vi "Calculate_Subtrack_Properties-1.vi"(6 "error IN":errorcluster, 7 "[IN] Areas particles\nPrimary Detected":dbl[][](array[numeric]), 8 "[IN] Primary \n(X,Y) Detected":dbl[][](array[numeric]), 9 "[IN] Subtrack":T1) -> (0 "error OUT":errorcluster, 1 "[OUT] Length of track":u8, 2 "[OUT] Areas":dbl[](array[numeric]), 3 "[OUT] dR (displ)":dbl[](array[numeric]))   [LabVIEW 2013]
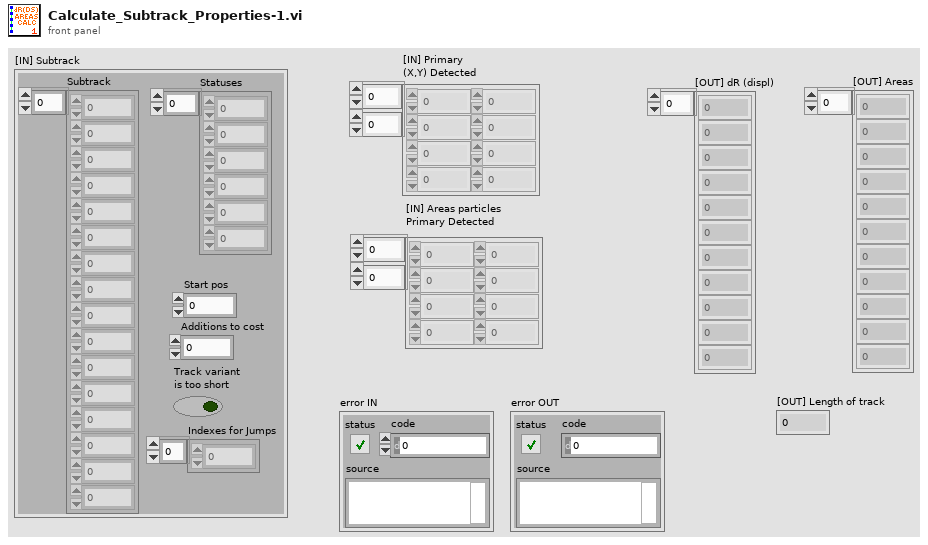
[diagram p1: front panel]
types:
  T1 = cluster{"Subtrack":dbl[], "Statuses":i16[], "Start pos":i32, "Additions to cost":i8, "Track variant \nis too short":bool, "Indexes for Jumps":i32[]}
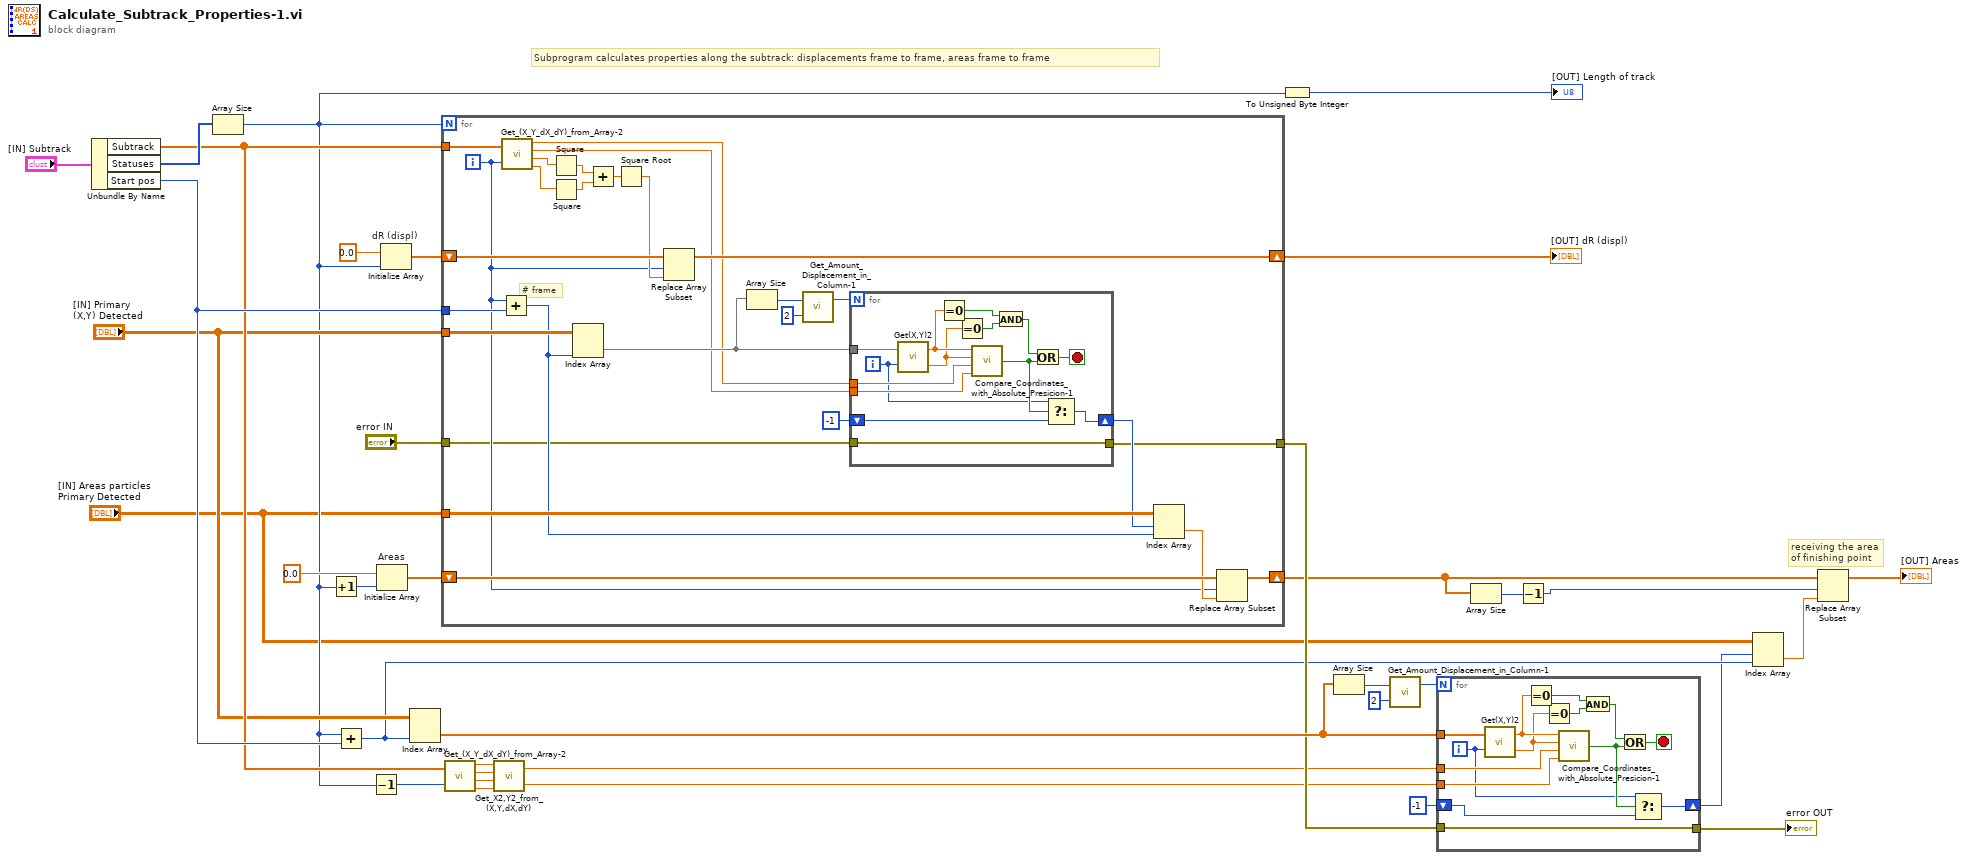
[diagram p0: block diagram]
diagram:
  # "receiving the area\nof finishing point"
  # "Subprogram calculates properties along the subtrack: displacements frame to frame, areas frame to frame"
  n1 = Unbundle By Name("[IN] Subtrack") -> ("Subtrack"=w25:dbl[], "Statuses"=w36:i16[], "Start pos"=w26:i32)
  n2 = Array Size(array=w36) -> (size(s)=w17:i32)
  n3 = Increment(x=w17) -> (x+1=w27:i32)
  n4 = Add(x=w17, y=w26) -> (x+y=w3:i32)
  n5 = Decrement(x=w17) -> (x-1=w16:i32)
  n6 = Initialize Array "Areas"(0.0 ("element"), w27) -> (w31:dbl[])
  n7 = Initialize Array "dR (displ)"(0.0 ("element"), w17) -> (w33:dbl[])
  n8 = Index Array(array="[IN] Primary \n(X,Y) Detected", index (col)=w3) -> (element=w19:dbl[])  [unwired: 1 in]
  n9 = for {
    N: w17 -> [_]
    tunnel: w25 -> [w63]
    shift-right: [w55] -> w29
    shift-left: w33 -> [w57]
    tunnel: "[IN] Primary \n(X,Y) Detected" -> [w54]
    tunnel: w26 -> [w53]
    tunnel: "[IN] Areas particles\nPrimary Detected" -> [w45]
    shift-right: [w39] -> w8
    shift-left: w31 -> [w42]
    tunnel: "error IN" -> [w38]
    tunnel: [w37] -> w18
    i -> [w40]
    # "# frame"
    n10 = Add(x=w40, y=w53) -> (x+y=w44:i32)
    n11 = call "Get_(X_Y_dX_dY)_from_Array-2.vi"("(X,Y,dX,dY)"=w63, "Index of Displacement"=w40) -> ("X"=w46:dbl, "Y"=w47:dbl, "dX"=w59:dbl, "dY"=w58:dbl)
    n12 = Square(x=w59) -> (x^2=w62:dbl)
    n13 = Square(x=w58) -> (x^2=w61:dbl)
    n14 = Index Array(array=w54, index (col)=w44) -> (element=w48:dbl[])  [unwired: 1 in]
    n15 = Add(x=w62, y=w61) -> (x+y=w60:dbl)
    n16 = Square Root(x=w60) -> (sqrt(x)=w56:dbl)
    n17 = Replace Array Subset(array=w57, new element=w56, index=w40) -> (w55:dbl[])
    n18 = Array Size(array=w48) -> (size(s)=w52:i32)
    n19 = call "Get_Amount_Displacement_in_Column-1.vi"("multiplier"=2, "# Rows"=w52) -> ("Displ amount"=w50:i32)  [unwired: 1 out]
    n20 = for {
      N: w50 -> [_]
      tunnel: w48 -> [w76]
      tunnel: w46 -> [w75]
      tunnel: w47 -> [w74]
      shift-right: [w65] -> w43
      shift-left: -1 -> [w66]
      tunnel: w38 -> [w64]
      tunnel: [w64] -> w37
      i -> [w67]
      stop <- w77 stop-if-true
      n21 = call "Get(X,Y)2.vi"("[IN] index of (X,Y)"=w67, "[IN] Array coordi\nnates (X,Y) in Frame"=w76) -> ("[OUT] Y"=w70:dbl, "[OUT] X"=w71:dbl)
      n22 = Equal To 0?(x=w71) -> (x = 0?=w73:bool)
      n23 = Equal To 0?(x=w70) -> (x = 0?=w72:bool)
      n24 = call "Compare_Coordinates_with_Absolute_Presicion-1.vi"("X 1"=w71, "Y 1"=w70, "X 2"=w75, "Y 2"=w74) -> ("[OUT] Same coordinates?"=w68:bool)  [unwired: 1 in]
      n25 = And(x=w73, y=w72) -> (x .and. y?=w69:bool)
      n26 = Or(x=w69, y=w68) -> (x .or. y?=w77:bool)
      n27 = Select(t=w67, s=w68, f=w66) -> (s? t:f=w65:i32)
    }
    n28 = Index Array(array=w45, index (row)=w43, index (col)=w44) -> (element=w41:dbl)
    n29 = Replace Array Subset(array=w42, new element=w41, index=w40) -> (w39:dbl[])
  }
  "[OUT] dR (displ)" <- w29
  n30 = call "Get_(X_Y_dX_dY)_from_Array-2.vi"("(X,Y,dX,dY)"=w25, "Index of Displacement"=w16) -> ("X"=w15:dbl, "Y"=w14:dbl, "dX"=w13:dbl, "dY"=w12:dbl)
  n31 = call "Get_X2,Y2_from_(X,Y,dX,dY).vi"("dY"=w12, "dX"=w13, "Y1"=w14, "X1"=w15) -> ("Y2 = (Y1+dY)"=w10:dbl, "X2 = (X1+dX)"=w11:dbl)
  n32 = To Unsigned Byte Integer(number=w17) -> (unsigned 8bit integer=→"[OUT] Length of track":u8)
  n33 = Array Size(array=w19) -> (size(s)=w23:i32)
  n34 = call "Get_Amount_Displacement_in_Column-1.vi"("multiplier"=2, "# Rows"=w23) -> ("Displ amount"=w21:i32)  [unwired: 1 out]
  n35 = for {
    N: w21 -> [_]
    tunnel: w19 -> [w90]
    tunnel: w11 -> [w89]
    tunnel: w10 -> [w88]
    shift-right: [w79] -> w2
    shift-left: -1 -> [w80]
    tunnel: w18 -> [w78]
    tunnel: [w78] -> w9
    i -> [w81]
    stop <- w91 stop-if-true
    n36 = call "Get(X,Y)2.vi"("[IN] index of (X,Y)"=w81, "[IN] Array coordi\nnates (X,Y) in Frame"=w90) -> ("[OUT] Y"=w84:dbl, "[OUT] X"=w85:dbl)
    n37 = Equal To 0?(x=w85) -> (x = 0?=w87:bool)
    n38 = Equal To 0?(x=w84) -> (x = 0?=w86:bool)
    n39 = call "Compare_Coordinates_with_Absolute_Presicion-1.vi"("X 1"=w85, "Y 1"=w84, "X 2"=w89, "Y 2"=w88) -> ("[OUT] Same coordinates?"=w82:bool)  [unwired: 1 in]
    n40 = And(x=w87, y=w86) -> (x .and. y?=w83:bool)
    n41 = Or(x=w83, y=w82) -> (x .or. y?=w91:bool)
    n42 = Select(t=w81, s=w82, f=w80) -> (s? t:f=w79:i32)
  }
  "error OUT" <- w9
  n43 = Array Size(array=w8) -> (size(s)=w7:i32)
  n44 = Decrement(x=w7) -> (x-1=w6:i32)
  n45 = Index Array(array="[IN] Areas particles\nPrimary Detected", index (row)=w2, index (col)=w3) -> (element=w1:dbl)
  n46 = Replace Array Subset(array=w8, new element=w1, index=w6) -> (→"[OUT] Areas":dbl[])
